vi "meth.StackDump.vi"(0 "class.GLue in":refnum<class "class.GLue.lvclass">, 11 "error in (no error)":errorcluster) -> (4 "class.GLue out":refnum<class "class.GLue.lvclass">, 8 "Stack":string[](array[string]), 15 "error out":errorcluster)   [LabVIEW 2014, in "GLue.lvlib" / "class.GLue.lvclass"]
uses:
  class.GLue.lvclass
  class.GLue.lvclass/class.GLue.ctl
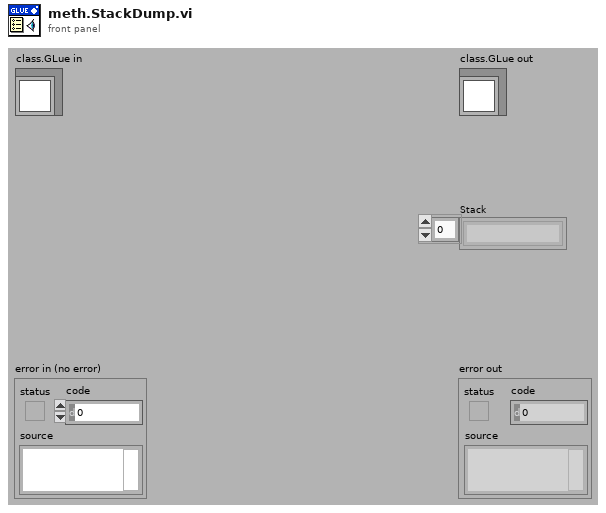
[diagram p1: front panel]
types:
  T1 = typedef "GLue.lvlib/class.GLue.lvclass/typedef.Types.ctl" = enum16{"Nil", "Bool", "LightUserData", "Number", "String", "Table", "Function", "UserData", "Thread"}
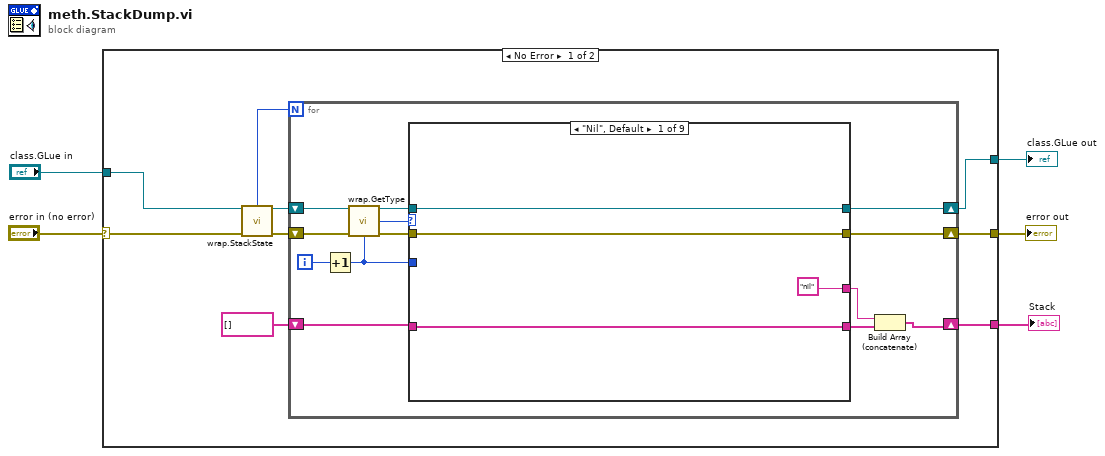
[diagram p0: block diagram]
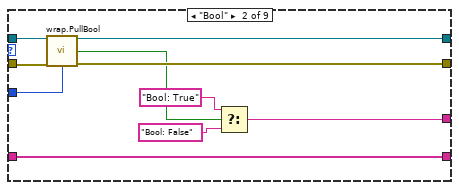
[diagram p2: hidden frame]
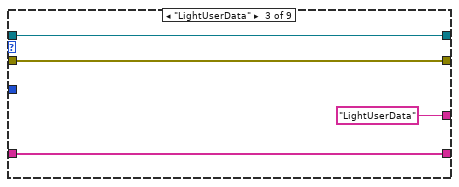
[diagram p3: hidden frame]
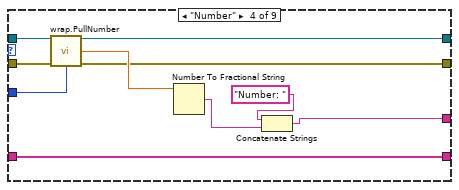
[diagram p4: hidden frame]
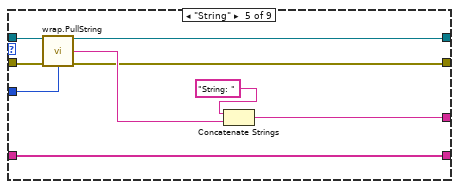
[diagram p5: hidden frame]
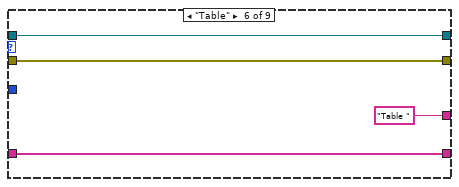
[diagram p6: hidden frame]
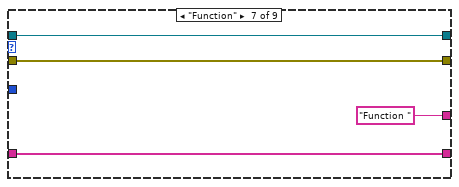
[diagram p7: hidden frame]
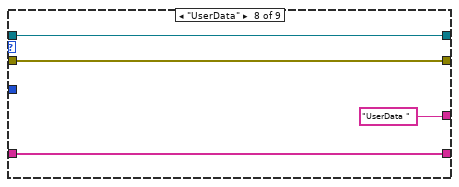
[diagram p8: hidden frame]
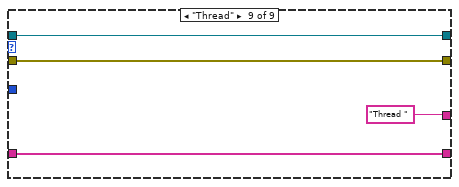
[diagram p9: hidden frame]
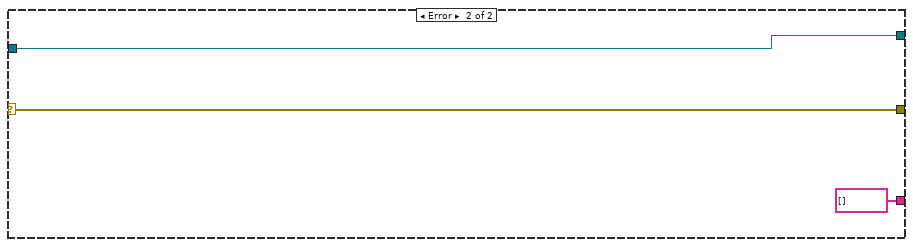
[diagram p10: hidden frame]
diagram:
  n1 = case shown="No Error" "error in (no error)" {
    selector: "error in (no error)" -> [w14 w83]
    tunnel: [w8 w83] -> w4
    tunnel: [w7 w82] -> w2
    tunnel: "class.GLue in" -> [w13 w82]
    tunnel: [w6 string[] [] ("Array")] -> w1
    frame No Error {
      n2 = call "wrap.StackState.vi"("class.GLue in"=w13, "error in (no error)"=w14) -> ("class.GLue out"=w12:refnum<class "class.GLue.lvclass">, "Size"=w10:i32, "error out"=w11:errorcluster)  [unwired: 10 in, 1 out]
      n3 = for {
        N: w10 -> [_]
        shift-right: [w17] -> w6
        shift-left: string[] [] ("Array") -> [w20]
        shift-right: [w19] -> w7
        shift-left: w12 -> [w26]
        shift-right: [w18] -> w8
        shift-left: w11 -> [w27]
        i -> [w25]
        n4 = Increment(x=w25) -> (x+1=w21:i32)
        n5 = call "wrap.GetType.vi"("class.GLue in"=w26, "error in (no error)"=w27, "Index"=w21) -> ("class.GLue out"=w23:refnum<class "class.GLue.lvclass">, "Type"=w22:T1, "error out"=w24:errorcluster)  [unwired: 10 in]
        n6 = case shown="\"Nil\", Default" w22 {
          tunnel: w24 -> [w30 w41 w44 w55 w63 w66 w70 w74 w78]
          tunnel: w23 -> [w31 w40 w45 w54 w62 w67 w71 w75 w79]
          tunnel: w20 -> [w29 w32 w43 w52 w64 w68 w72 w76 w80]
          tunnel: w21 -> [_ w39 _ w53 w61 _ _ _ _]
          tunnel: [w29 w32 w43 w52 w64 w68 w72 w76 w80] -> w16
          tunnel: [w31 w38 w45 w49 w57 w67 w71 w75 w79] -> w19
          tunnel: [w30 w37 w44 w50 w58 w66 w70 w74 w78] -> w18
          tunnel: ["nil" w33 "LightUserData" w46 w56 "Table " "Function " "UserData " "Thread "] -> w15
          frame "Nil", Default {
          }
          frame "Bool" {
            n7 = call "wrap.PullBool.vi"("class.GLue in"=w40, "error in (no error)"=w41, "Index"=w39) -> ("class.GLue out"=w38:refnum<class "class.GLue.lvclass">, "Boolean"=w36:bool, "error out"=w37:errorcluster)  [unwired: 10 in]
            n8 = Select(t="Bool: True", s=w36, f="Bool: False") -> (s? t:f=w33:string)
          }
          frame "LightUserData" {
          }
          frame "Number" {
            n9 = call "wrap.PullNumber.vi"("class.GLue in"=w54, "error in (no error)"=w55, "Index"=w53) -> ("class.GLue out"=w49:refnum<class "class.GLue.lvclass">, "Number"=w51:dbl, "error out"=w50:errorcluster)  [unwired: 10 in]
            n10 = Number To Fractional String(number=w51) -> (F-format string=w47:string)  [unwired: 3 in]
            n11 = Concatenate Strings("Number: ", w47) -> (w46:string)
          }
          frame "String" {
            n12 = call "wrap.PullString.vi"("class.GLue in"=w62, "error in (no error)"=w63, "Index"=w61) -> ("class.GLue out"=w57:refnum<class "class.GLue.lvclass">, "String"=w59:string, "error out"=w58:errorcluster)  [unwired: 10 in]
            n13 = Concatenate Strings("String: ", w59) -> (w56:string)
          }
          frame "Table" {
          }
          frame "Function" {
          }
          frame "UserData" {
          }
          frame "Thread" {
          }
        }
        n14 = Build Array (concatenate)(w15, w16) -> (w17:string[])
      }
    }
    frame Error {
    }
  }
  "error out" <- w4
  "class.GLue out" <- w2
  "Stack" <- w1
